vi "WT500 General Setup.vi"(0 "VISA Refnum in":refnum<visa-resource-name>, 2 "Wiring (0: 1P2W, 1P2W, 1P2W)":T1=1 items=["1P2W, 1P2W, 1P2W", "1P3W, 1P2W", "3P3W, 1P2W", "1P2W, 1P3W", "1P2W, 3P3W", "3P4W", "3V3A"], 3 "V Range (8: 1000V)":u16(ring)=6 items=["AUTO", "15", "30", "60", "100", "150", "300", "600", "1000", "7.5", "15", "30", "50", "75", "150", "300", "500"], 5 "error in (no error)":errorcluster, 6 "Element (0: All)":u16(ring) items=["All", "Element 1", "Element 2", "Element 3", "Sigma"], 7 "Display Format":u16(ring) items=["Numeric", "Wave", "Bar", "Vector", "Trend"], 8 "Update Rate (3: 500ms)":u16(ring)=2 items=["-", "100ms", "200ms", "500ms", "1s", "2s", "5s"], 9 "I Range (7: 40A)":u16(ring)=7 items=["AUTO", "500 mA", "1 A", "2 A", "5 A", "10 A", "20 A", "40 A", "S-AUTO", "50 mV", "100 mV", "200 mV", "500 mV", "1 V", "2 V", "5 V", "10 V", "250 mA", "500 mA", "1 A", "2.5 A", "5 A", "10 A", "20 A", "25 mV", "50 mV", "100 mV", "250 mV", "500 mV", "1 V", "2.5 V", "5 V"], 11 "Reset Wh":bool=TRUE, 12 "Crest Factor (0: 3)":u16(ring) items=["3", "6"]) -> (10 "Array of Measurements":u16[](array[numeric]), 14 "VISA Refnum out":refnum<visa-resource-name>, 16 "Instrument ID":string, 17 "Array Locations":u16[](array[numeric]), 19 "error out":errorcluster)   [LabVIEW 2016]
uses:
  Type Definitions/WT500 Wiring Control.ctl
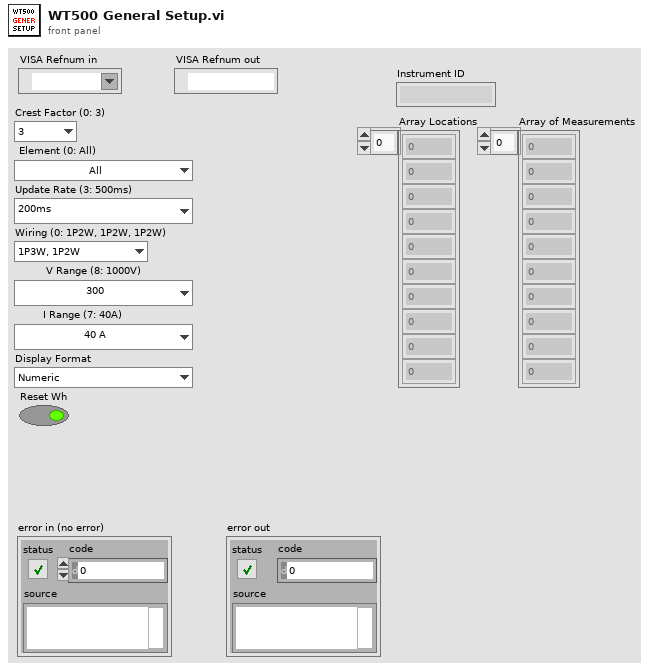
[diagram p1: front panel]
types:
  T1 = typedef "WT500 Wiring Control.ctl" = u16
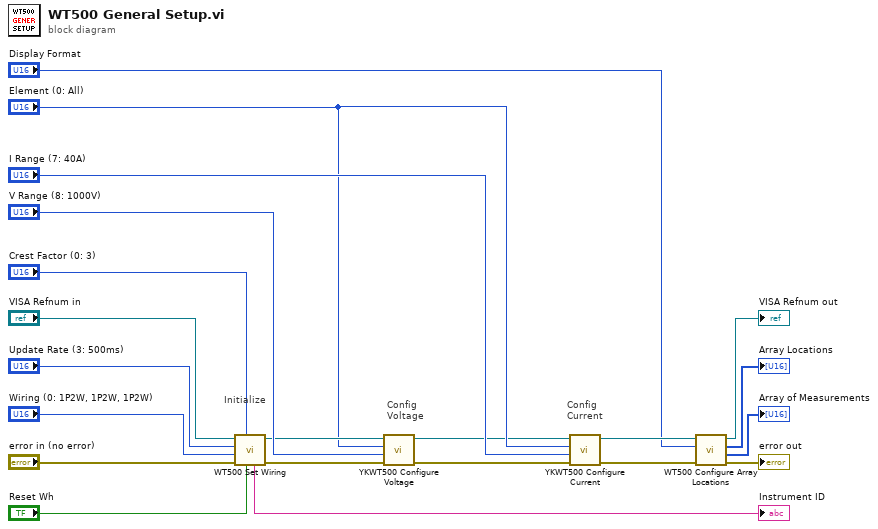
[diagram p0: block diagram]
diagram:
  # "Config\nCurrent"
  # "Config\nVoltage"
  # "Initialize"
  n1 = call "WT500 Set Wiring.vi"("Reset Wh"="Reset Wh", "Crest Factor (0: 3)"="Crest Factor (0: 3)", "error in (no error)"="error in (no error)", "Wiring (0: 1P2W, 1P2W, 1P2W)"="Wiring (0: 1P2W, 1P2W, 1P2W)", "Update Rate (3: 500ms)"="Update Rate (3: 500ms)", "VISA Refnum in"="VISA Refnum in") -> ("error out"=w6:errorcluster, "VISA Refnum out"=w7:refnum<visa-resource-name>, "Instrument ID"=→"Instrument ID":string)  [unwired: 3 in]
  n2 = call "YKWT500 Configure Voltage.vi"("error in (no error)"=w6, "Voltage Range (8: 1000V)"="V Range (8: 1000V)", "Element (0: All)"="Element (0: All)", "VISA resource name"=w7) -> ("error out"=w1:errorcluster, "VISA resource name out"=w2:refnum<visa-resource-name>)  [unwired: 6 in]
  n3 = call "YKWT500 Configure Current.vi"("error in (no error)"=w1, "Current Range (7: 40A)"="I Range (7: 40A)", "Element (0: All)"="Element (0: All)", "VISA resource name"=w2) -> ("error out"=w20:errorcluster, "VISA resource name out"=w21:refnum<visa-resource-name>)  [unwired: 6 in]
  n4 = call "WT500 Configure Array Locations.vi"("error in (no error)"=w20, "Display Format"="Display Format", "VISA Refnum in"=w21) -> ("error out"=→"error out":errorcluster, "Array of Measurements"=→"Array of Measurements":u16[], "Array Locations"=→"Array Locations":u16[], "VISA Refnum out"=→"VISA Refnum out":refnum<visa-resource-name>)  [unwired: 5 in]
